vi "Constructor with Impulse Reference.vi"(11 "Impulse Object Reference":T1) -> (3 "Impulse Manager.lvclass":refnum<class "Impulse Manager.lvclass">)   [LabVIEW 2016, in "Impulse Manager.lvclass"]
uses:
  Impulse Manager.lvclass
  Impulse Data/Instance handle.ctl
  Impulse Data/Impulse Data.lvclass
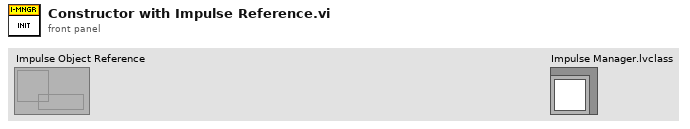
[diagram p1: front panel]
types:
  T1 = typedef "Impulse Data.lvclass/Instance handle.ctl" = refnum<data-value>
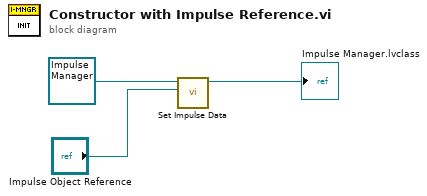
[diagram p0: block diagram]
diagram:
  n1 = call-dynamic "Set Impulse Data.vi"("Impulse Object Reference"="Impulse Object Reference", "Impulse Manager in"=refnum<class "Impulse Manager.lvclass"> refnum ("Impulse Manager.lvclass")) -> ("Impulse Manager out"=→"Impulse Manager.lvclass":refnum<class "Impulse Manager.lvclass">)  [unwired: 8 in, 1 out]
